vi "Read VI Refnum.vi"(8 "error in (no error)":errorcluster, 11 "Module Data In":refnum<class "Rename.lvclass">) -> (0 "error out":errorcluster, 2 "VI Refnum":refnum<vi>, 3 "Module Data Out":refnum<class "Rename.lvclass">)   [LabVIEW 2015, in "Generic Module Library.lvlib" / "Template G_Module.lvlib" / "Rename.lvclass"]
uses:
  Rename.lvclass
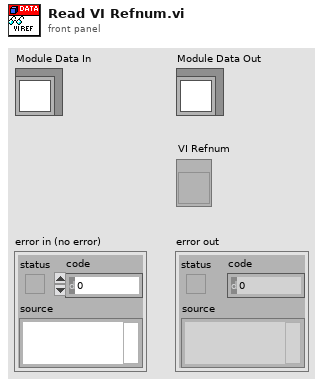
[diagram p1: front panel]
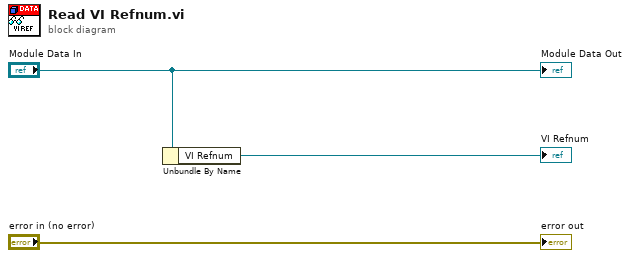
[diagram p0: block diagram]
diagram:
  n1 = Unbundle By Name("Module Data In") -> ("VI Refnum"=→"VI Refnum":refnum<vi>)
  "error out" <- "error in (no error)"
  "Module Data Out" <- "Module Data In"
